vi "Programmed Move.vi"(8 "error in (no error)":errorcluster, 9 "Index 2":u16, 10 "Index":i32, 11 "VacuumLines in":refnum<class "VacuumLines.lvclass">) -> (0 "error out":errorcluster, 2 "Target pos":dbl, 3 "VacuumLines out":refnum<class "VacuumLines.lvclass">)   [LabVIEW 2016, in "Hardware.lvlib" / "VacuumLine.lvlib" / "VacuumLines.lvclass"]
uses:
  <userlib>/Common Components/Hardware/Abstract System/VacuumLine/VacuumLines/VacuumLines.lvclass
  <userlib>/Common Components/Hardware/Abstract System/VacuumLine/VacuumLines/VacuumLines.lvclass/VacuumLines.ctl
  <userlib>/Common Components/Hardware/Abstract System/VacuumLine/VacuumLine/VacuumLine.lvclass/VacuumLine.ctl
  <userlib>/Common Components/Hardware/Abstract System/VacuumLine/VacuumLine/VacuumLine.lvclass
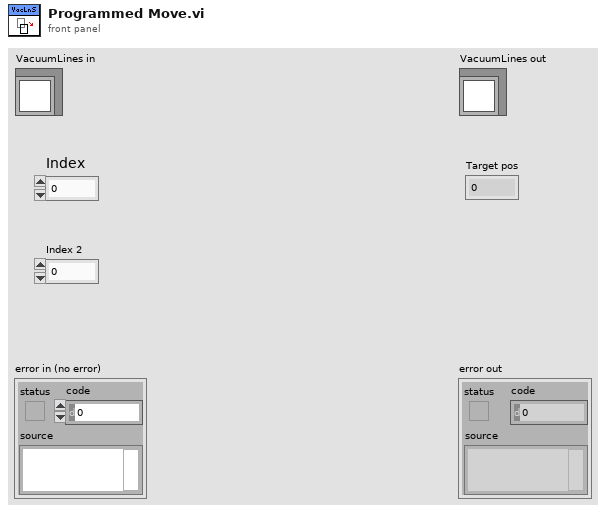
[diagram p1: front panel]
types:
  T1 = typedef "Hardware.lvlib/VacuumLine.lvlib/VacuumLine.lvclass/Button Config Cluster.ctl" = cluster{"Enabled?":bool, "Text on button":string, "Target pos":dbl}
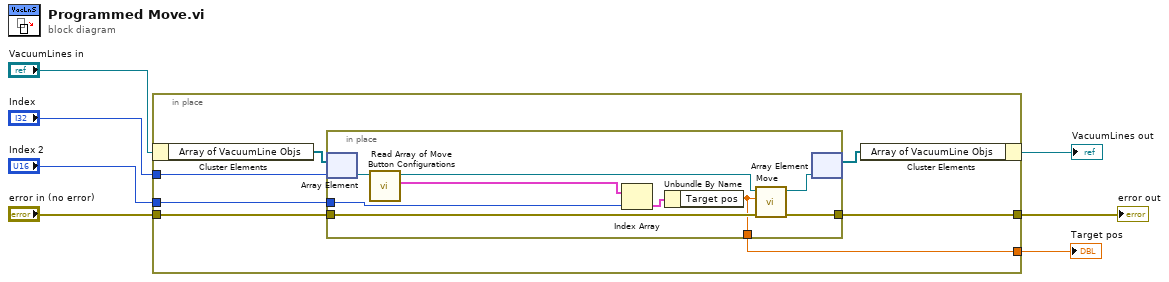
[diagram p0: block diagram]
diagram:
  n1 = in-place {
    in-place-border: "Index" -> [w13]
    in-place-border: "error in (no error)" -> [w11]
    in-place-border: [w10] -> w3
    in-place-border: "Index 2" -> [w9]
    in-place-border: [w8] -> w1
    n2 = in-place-cluster #1("VacuumLines in") -> ("Array of VacuumLine Objs"=w14:refnum<class "VacuumLine.lvclass">[])
    n3 = in-place {
      in-place-border: w11 -> [w22]
      in-place-border: [w21] -> w10
      in-place-border: w9 -> [w17]
      in-place-border: [w15] -> w8
      n4 = in-place-array #2(w14, w13) -> (w20:refnum<class "VacuumLine.lvclass">)
      n5 = call <userlib>:"Read Array of Move Button Configurations.vi"("VacuumLine in"=w20) -> ("Array of Move Button Configurations"=w18:T1[], "VacuumLine out"=w19:refnum<class "VacuumLine.lvclass">)  [unwired: 9 in]
      n6 = Index Array(array=w18, index=w17) -> (element=w16:T1)
      n7 = Unbundle By Name(w16) -> ("Target pos"=w15:dbl)
      n8 = call <userlib>:"Move.vi"("error in (no error)"=w22, "target pos"=w15, "VacuumLine in"=w19) -> ("error out"=w21:errorcluster, "VacuumLine out"=w23:refnum<class "VacuumLine.lvclass">)  [unwired: 7 in]
      n9 = in-place-array #2(w23) -> (w12:refnum<class "VacuumLine.lvclass">[])  [unwired: 1 out]
    }
    n10 = in-place-cluster #1("Array of VacuumLine Objs"=w12) -> (→"VacuumLines out":refnum<class "VacuumLines.lvclass">)
  }
  "error out" <- w3
  "Target pos" <- w1
